vi "LEUI_Create_Blink_Expected_LEDs.vi"(7 "Boolean":bool) -> (8 "Expected LEDs Out":T1)   [LabVIEW 2016, in "TLMB.lvlib"]
uses:
  Projects/TLMB.lvlib
  controls/LEUI_LEDs.ctl
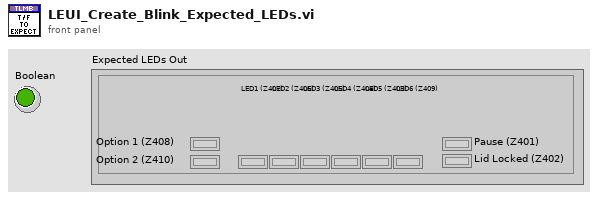
[diagram p1: front panel]
types:
  T1 = typedef "TLMB.lvlib/LEUI_LEDs.ctl" = cluster{"Pause (Z401)":bool, "Lid Locked (Z402)":bool, "LED1 (Z407)":bool, "LED2 (Z406)":bool, "LED3 (Z405)":bool, "LED4 (Z404)":bool, "LED5 (Z403)":bool, "LED6 (Z409)":bool, "Option 1 (Z408)":bool, "Option 2 (Z410)":bool}
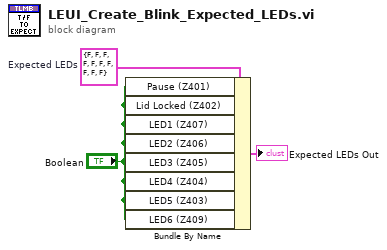
[diagram p0: block diagram]
diagram:
  w3 = T1 {"Pause (Z401)"=FALSE, "Lid Locked (Z402)"=FALSE, "LED1 (Z407)"=FALSE, "LED2 (Z406)"=FALSE, "LED3 (Z405)"=FALSE, "LED4 (Z404)"=FALSE, "LED5 (Z403)"=FALSE, "LED6 (Z409)"=FALSE, "Option 1 (Z408)"=FALSE, "Option 2 (Z410)"=FALSE}  # Expected LEDs
  n1 = Bundle By Name(cluster=w3, "Pause (Z401)"="Boolean", "Lid Locked (Z402)"="Boolean", "LED1 (Z407)"="Boolean", "LED2 (Z406)"="Boolean", "LED3 (Z405)"="Boolean", "LED4 (Z404)"="Boolean", "LED5 (Z403)"="Boolean", "LED6 (Z409)"="Boolean") -> (→"Expected LEDs Out":T1)
